vi "Update_odour_components.vi"(6 "Position":T3, 9 "Bounds":T4, 10 "Coords":T2, 11 "Odour bottles in":T1(array[cluster])) -> (0 "accept":bool, 3 "Odou bottle out":T1(array[cluster]))   [LabVIEW 2016]
uses:
  <vilib>/Utility/miscctls.llb/LVBoundsTypeDef.ctl
  <vilib>/Utility/miscctls.llb/LVPositionTypeDef.ctl
  <vilib>/Utility/miscctls.llb/LVPoint32TypeDef.ctl
  <vilib>/Analysis/NI_AALBase.lvlib
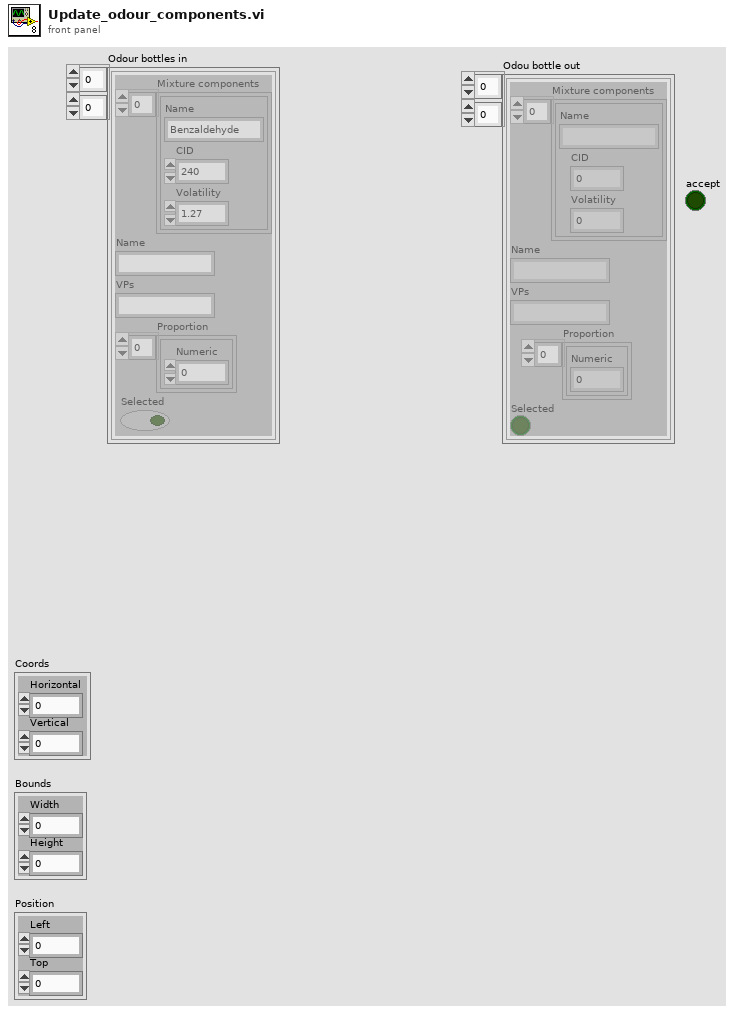
[diagram p1: front panel]
types:
  T1 = cluster{"Mixture components":cluster{"Name":string, "CID":i32, "Volatility":dbl}[], "Name":string, "VPs":string, "Proportion":cluster{"Numeric":dbl}[], "Selected":bool}[][]
  T2 = typedef "LVPoint32TypeDef.ctl" = cluster{"Horizontal":i32, "Vertical":i32}
  T3 = typedef "LVPositionTypeDef.ctl" = cluster{"Left":i32, "Top":i32}
  T4 = typedef "LVBoundsTypeDef.ctl" = cluster{"Width":u32, "Height":u32}
  T5 = cluster{"Name":string, "CID":i32, "Volatility":dbl}
  T6 = cluster{"Mixture components":cluster{"Name":string, "CID":i32, "Volatility":dbl}[], "Name":string, "VPs":string, "Proportion":cluster{"Numeric":dbl}[], "Selected":bool}
  T7 = cluster{"Name":string, "CID":i32, "Volatility":dbl}[]
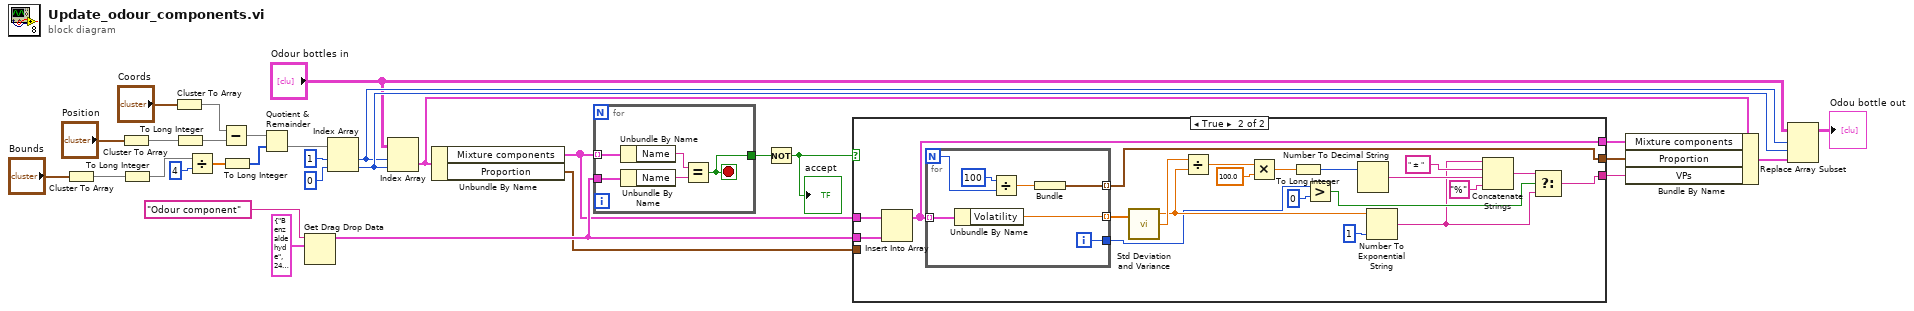
[diagram p0: block diagram]
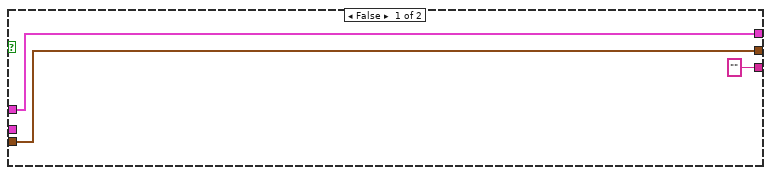
[diagram p2: hidden frame]
diagram:
  n1 = Cluster To Array(cluster="Bounds") -> (array=w14:u32[])
  n2 = Cluster To Array(cluster="Position") -> (array=w12:i32[])
  n3 = To Long Integer(number=w14) -> (32bit integer=w15:i32[])
  n4 = Cluster To Array(cluster="Coords") -> (array=w16:i32[])
  n5 = To Long Integer(number=w12) -> (32bit integer=w17:i32[])
  n6 = Divide(x=w15, y=4) -> (x/y=w23:dbl[])
  n7 = Subtract(x=w16, y=w17) -> (x-y=w18:i32[])
  n8 = To Long Integer(number=w23) -> (32bit integer=w24:i32[])
  n9 = Quotient & Remainder(x=w18, y=w24) -> (floor(x/y)=w20:i32[])  [unwired: 1 out]
  n10 = Get Drag Drop Data(8:T5 {"Name"="Benzaldehyde", "CID"=240, "Volatility"=1.27} ("Odour component"), 9:"Odour component" ("data name")) -> (3:w9:T5)  [unwired: 1 in, 1 out]
  n11 = Index Array(array=w20, index #1=1 ("index"), index #2=0 ("index")) -> (element #1=w27:i32, element #2=w28:i32)
  n12 = Index Array(array="Odour bottles in", index (row)=w27, index (col)=w28) -> (element=w26:T6)
  n13 = Unbundle By Name(w26) -> ("Mixture components"=w8:T7, "Proportion"=w5:cluster{"Numeric":dbl}[])
  n14 = for {
    tunnel: w8 -> [w36] mode=indexing
    tunnel: w9 -> [w34]
    tunnel: [w32] -> w7
    stop <- w32 stop-if-true
    n15 = Unbundle By Name(w36) -> ("Name"=w35:string)
    n16 = Unbundle By Name(w34) -> ("Name"=w33:string)
    n17 = Equal?(x=w35, y=w33) -> (x = y?=w32:bool)
  }
  n18 = Not(x=w7) -> (.not. x?=w6:bool)
  "accept" <- w6
  n19 = case shown="True" w6 {
    tunnel: [w39 w60] -> w31
    tunnel: [w38 w59] -> w30
    tunnel: w9 -> [_ w58]
    tunnel: w8 -> [w38 w57]
    tunnel: w5 -> [w39 _]
    tunnel: ["" w41] -> w1
    frame False {
    }
    frame True {
      n20 = Insert Into Array(array=w57, new element=w58) -> (w59:T7)  [unwired: 1 in]
      n21 = for {
        N -> [w65]
        tunnel: w59 -> [w63] mode=indexing
        tunnel: [w67] -> w60 mode=indexing
        tunnel: [w62] -> w56 mode=indexing
        tunnel: [w61] -> w45
        i -> [w61]
        n22 = Unbundle By Name(w63) -> ("Volatility"=w62:dbl)
        n23 = Divide(x=100 ("y"), y=w65) -> (x/y=w64:dbl)
        n24 = Bundle(w64) -> (w67:cluster{dbl})  [unwired: 1 in]
      }
      n25 = call <vilib>:"Std Deviation and Variance.vi"("X"=w56) -> ("mean"=w47:dbl, "standard deviation"=w55:dbl)  [unwired: 1 in, 1 out]
      n26 = Divide(x=w55, y=w47) -> (x/y=w53:dbl)
      n27 = Multiply(x=w53, y=100.0) -> (x*y=w52:dbl)
      n28 = To Long Integer(number=w52) -> (32bit integer=w49:i32)
      n29 = Greater?(x=w45, y=0) -> (0:w43:bool)
      n30 = Number To Decimal String(number=w49) -> (decimal integer string=w50:string)  [unwired: 1 in]
      n31 = Number To Exponential String(number=w47, precision (6)=i16 1) -> (E-format string=w40:string)  [unwired: 2 in]
      n32 = Concatenate Strings(w40, " ± " ("string"), w50, "%" ("string")) -> (w42:string)
      n33 = Select(t=w42, s=w43, f=w40) -> (s? t:f=w41:string)
    }
  }
  n34 = Bundle By Name(cluster=w26, "Mixture components"=w30, "Proportion"=w31, "VPs"=w1) -> (w29:T6)
  n35 = Replace Array Subset(array="Odour bottles in", new element=w29, index (row)=w27, index (col)=w28) -> (→"Odou bottle out":T1)
